vi "rounding_number.vi"(9 "decimal Places":dbl, 11 "Numeric":dbl) -> (3 "rounded number":dbl)   [LabVIEW 2014]
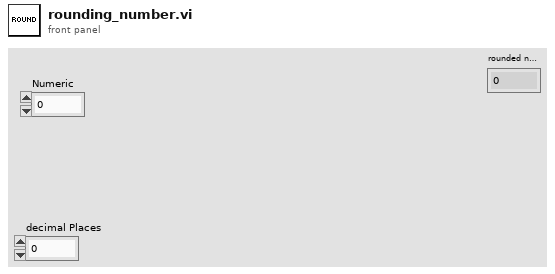
[diagram p1: front panel]
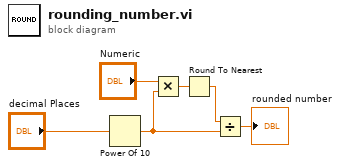
[diagram p0: block diagram]
diagram:
  n1 = Power Of 10(x="decimal Places") -> (10^x=w2:dbl)
  n2 = Multiply(x="Numeric", y=w2) -> (x*y=w4:dbl)
  n3 = Round To Nearest(number=w4) -> (nearest integer value=w3:dbl)
  n4 = Divide(x=w3, y=w2) -> (x/y=→"rounded number":dbl)
